vi "SetOutputeEnableState.vi"(8 "Error In":errorcluster, 10 "Enabled?":bool, 11 "Keithley 6482 In":refnum<visa-resource-name>) -> (0 "Error Out":errorcluster, 3 "Keithley 6482 Out":refnum<visa-resource-name>)   [LabVIEW 2014, in "Keithley-6482-Visa.lvlib"]
uses:
  Keithley-6482-Visa.lvlib
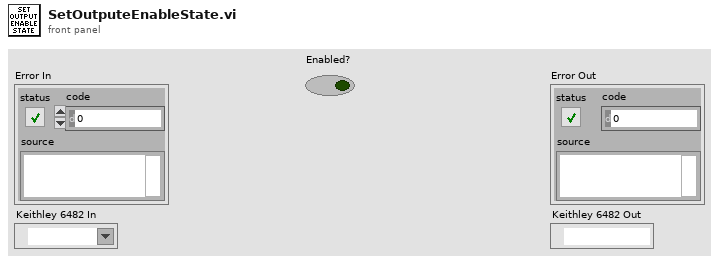
[diagram p1: front panel]
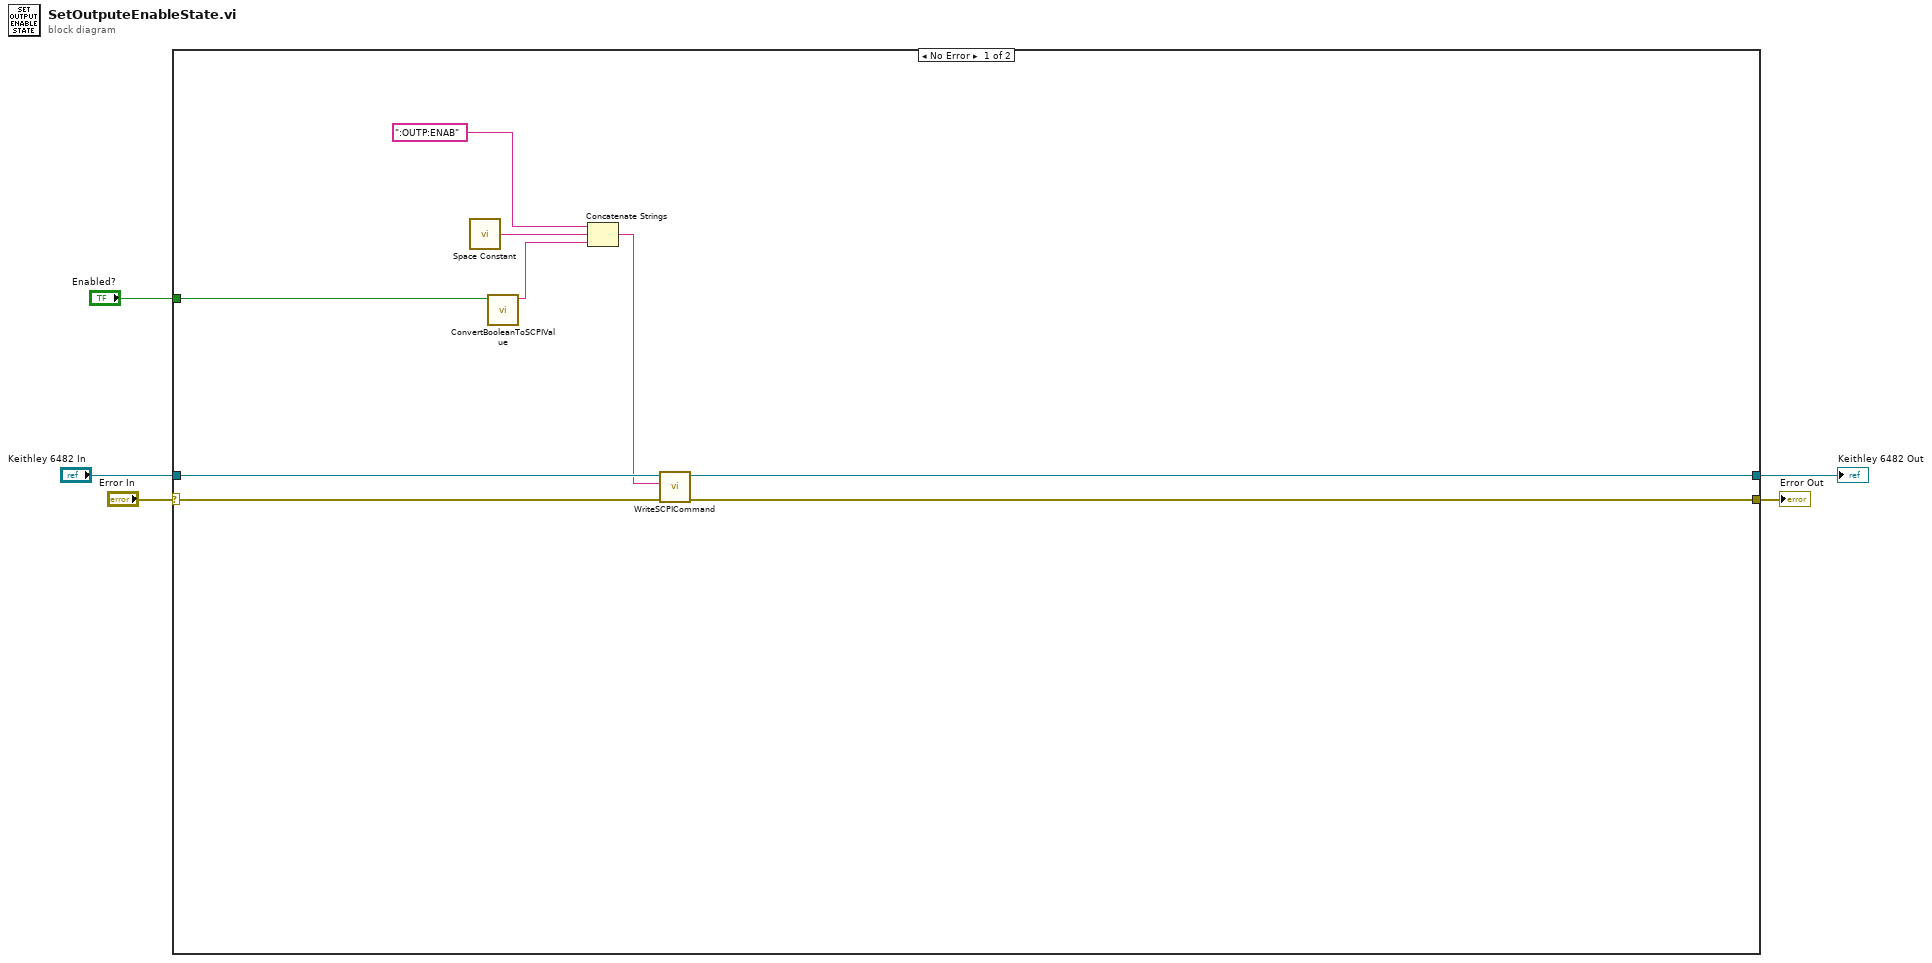
[diagram p0: block diagram]
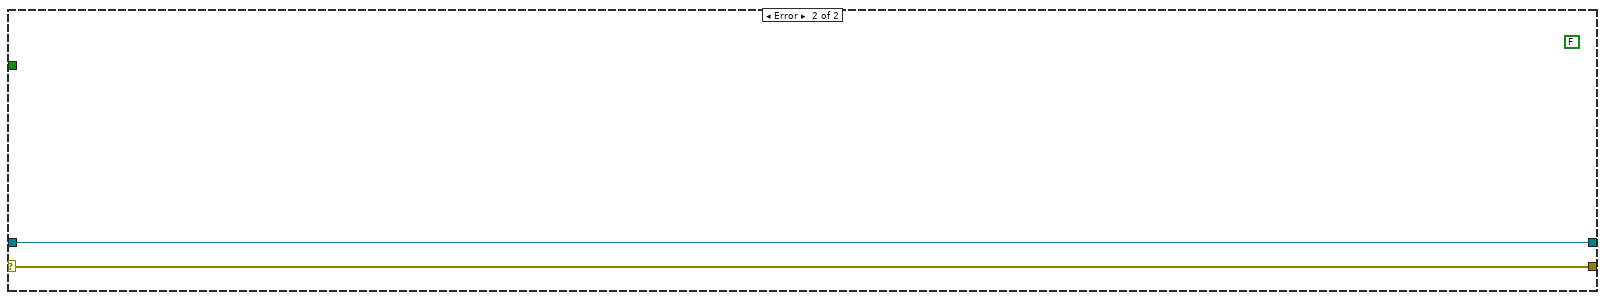
[diagram p2: hidden frame]
diagram:
  n1 = case shown="No Error" "Error In" {
    selector: "Error In" -> [w13 w15]
    tunnel: [w10 w15] -> w4
    tunnel: [w11 w16] -> w3
    tunnel: "Keithley 6482 In" -> [w14 w16]
    tunnel: "Enabled?" -> [w8 _]
    frame No Error {
      n2 = call <vilib>:"Space Constant.vi"() -> ("String"=w9:string)
      n3 = call "ConvertBooleanToSCPIValue.vi"("Boolean"=w8) -> ("SCPI Value"=w7:string)  [unwired: 10 in]
      n4 = Concatenate Strings(":OUTP:ENAB", w9, w7) -> (w6:string)
      n5 = call "WriteSCPICommand.vi"("Error In"=w13, "SCPI Command"=w6, "Keithley 6482 In"=w14) -> ("Error Out"=w10:errorcluster, "Keithley 6482 Out"=w11:refnum<visa-resource-name>)  [unwired: 7 in]
    }
    frame Error {
      (unwired) FALSE ("Boolean")
    }
  }
  "Error Out" <- w4
  "Keithley 6482 Out" <- w3
